vi "elaborate.vi"(0 "reference in":refnum<class "subject.lvclass">, 1 "phase":T2, 2 "threshold":dbl format="%#_13g", 3 "Width":i32, 4 "resultsType":T1, 5 "error in (no error)":errorcluster) -> (14 "reference out":refnum<class "subject.lvclass">, 19 "error out":errorcluster)   [LabVIEW 2015, in "subject.lvclass"]
uses:
  subject.lvclass
  phase.ctl
  resultsType.ctl
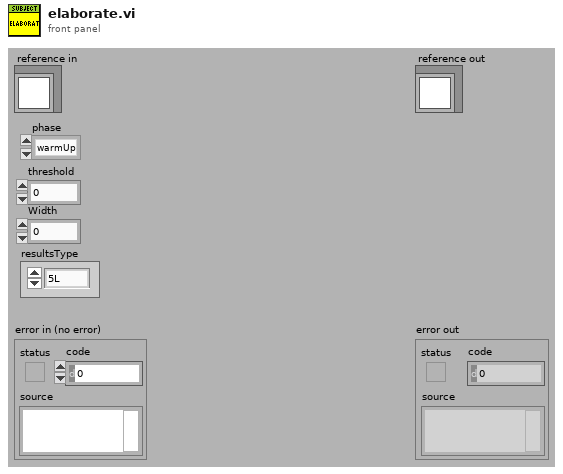
[diagram p1: front panel]
types:
  T1 = typedef "subject.lvclass/resultsType.ctl" = enum16{"5L", "15%", "User Selection"}
  T2 = typedef "subject.lvclass/phase.ctl" = enum16{"warmUp", "userSelection", "Exercise"}
  T3 = typedef "subject.lvclass/ObjectAttributesRef.ctl" = refnum<data-value>
  T4 = typedef "subject.lvclass/ObjectAttributes.ctl" = cluster{"MyAttribute":dbl, "data":cluster{"Ve_warm":dbl[], "time_warm":dbl[], "name":string, "phase":dbl[], "VCO2":dbl[], "VO2":dbl[], "PetCO2":dbl[], "RQ":dbl[], "HR":dbl[], "Ve_warm_inter":dbl[], "time_warm_inter":dbl[], "Ve_exer":dbl[], "time_exer":dbl[], "Ve_exer_inter":dbl[], "time_exer_inter":dbl[], "Ve":dbl[], "time":dbl[], "Ve_exer_inter_filtered":dbl[], "Ve_warm_inter_filtered":dbl[]}, "results_5l":cluster{"EOV":bool, "osci_amplitude":dbl[], "osci_width":dbl[], "peak_location":dbl[], "threshold":dbl, "width":i32}, "results_15percent":cluster{"EOV":bool, "osci_amplitude":dbl[], "osci_width":dbl[], "peak_location":dbl[], "threshold":dbl, "width":i32}, "supportData":cluster{"peaksAmplitude":dbl[], "iPeaksLocation":dbl[], "valesAmplitude":dbl[], "iValesLocation":dbl[], "threshold":dbl, "meanAmpl_warm":i32, "#_peaks":i32, "width":i32}, "results_user_selection":cluster{"EOV":bool, "osci_amplitude":dbl[], "osci_width":dbl[], "peak_location":dbl[], "threshold":dbl, "width":i32}, "results_warm_up":cluster{"EOV":bool, "osci_amplitude":dbl[], "osci_width":dbl[], "peak_location":dbl[], "threshold":dbl, "width":i32}}
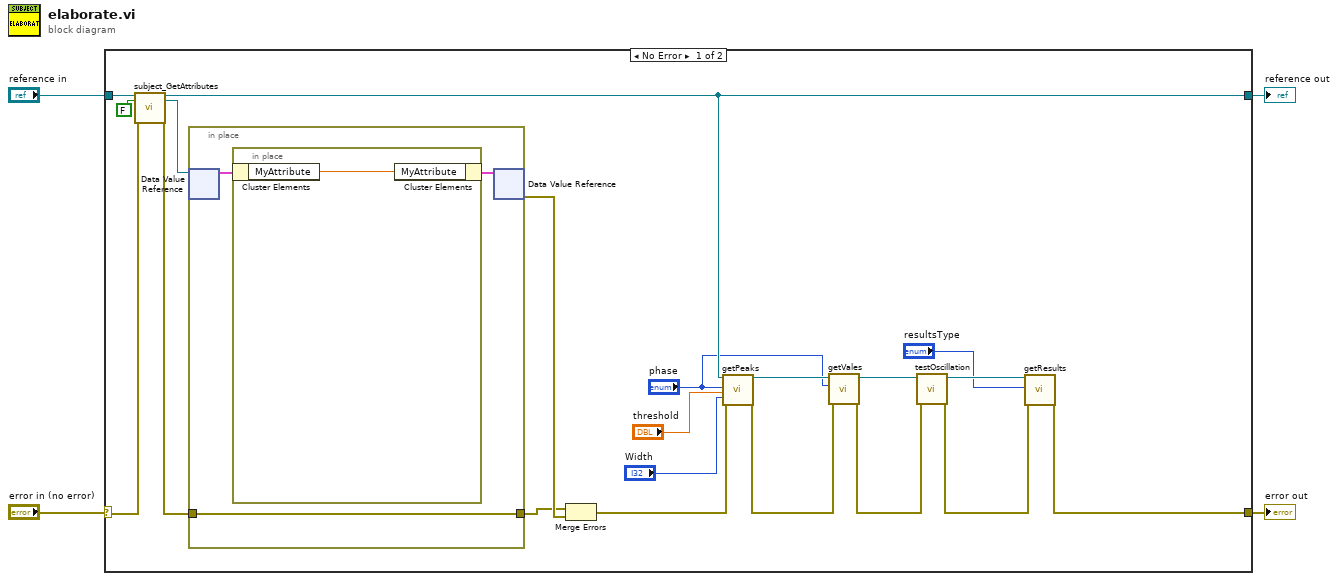
[diagram p0: block diagram]
diagram:
  n1 = case shown="No Error" "error in (no error)" {
    selector: "error in (no error)" -> [w20 w30]
    tunnel: [w16 w30] -> w3
    tunnel: [w15 w29] -> w1
    tunnel: "reference in" -> [w22 w29]
    frame No Error {
      n2 = call "subject_GetAttributes.vi"("reference in"=w22, "return data? (T)"=FALSE, "error in (no error)"=w20) -> ("reference out"=w15:refnum<class "subject.lvclass">, "attributes ref"=w18:T3, "error out"=w19:errorcluster)  [unwired: 13 in, 1 out]
      n3 = in-place {
        in-place-border: w19 -> [w25]
        in-place-border: [w25] -> w23
        n4 = in-place-dvr #1(w18) -> (w26:T4)  [unwired: 1 out]
        n5 = in-place {
          n6 = in-place-cluster #2(w26) -> ("MyAttribute"=w28:dbl)
          n7 = in-place-cluster #2("MyAttribute"=w28) -> (w27:T4)
        }
        n8 = in-place-dvr #1(w27) -> (w24:errorcluster)  [unwired: 1 out]
      }
      n9 = Merge Errors(w23, w24) -> (w17:errorcluster)
      n10 = call "getPeaks.vi"("reference in"=w15, "phase"="phase", "threshold"="threshold", "Width"="Width", "error in (no error)"=w17) -> ("reference out"=w14:refnum<class "subject.lvclass">, "error out"=w9:errorcluster)  [unwired: 13 in]
      n11 = call "getVales.vi"("error in (no error)"=w9, "phase"="phase", "reference in"=w14) -> ("error out"=w10:errorcluster, "reference out"=w13:refnum<class "subject.lvclass">)  [unwired: 7 in]
      n12 = call "testOscillation.vi"("error in (no error)"=w10, "reference in"=w13) -> ("error out"=w11:errorcluster, "reference out"=w12:refnum<class "subject.lvclass">)  [unwired: 8 in]
      n13 = call "getResults.vi"("reference in"=w12, "resultsType"="resultsType", "error in (no error)"=w11) -> ("error out"=w16:errorcluster)  [unwired: 15 in, 1 out]
    }
    frame Error {
    }
  }
  "error out" <- w3
  "reference out" <- w1
